vi "Asynchronous Logging Loop.vi"(10 "Input Data":T8 {"File Logging Specs"."File Node Ref" format="%.0x"}) -> ()   [LabVIEW 2027, in "Embedded Data Logger Engine.lvlib"]
uses:
  Embedded Data Logger Engine.lvlib
  File Logging Specification.ctl
  Group Logging Specification.ctl
  Group Buffer Data.ctl
  Property Specification.ctl
  <vilib>/NI VeriStand/Custom Device API/Custom Device Item Ref.ctl
  Shared/Segment Files By.ctl
  Logging State.ctl
  Asynchronous Logging Loop State.ctl
  Add to Flushed Data Size.vi
  Scripting/Embedded Data Logger Scripting.lvlib
  <vilib>/NI VeriStand/Custom Device API/Custom Device API.lvlib
  Shared/Embedded Data Logger Shared.lvlib
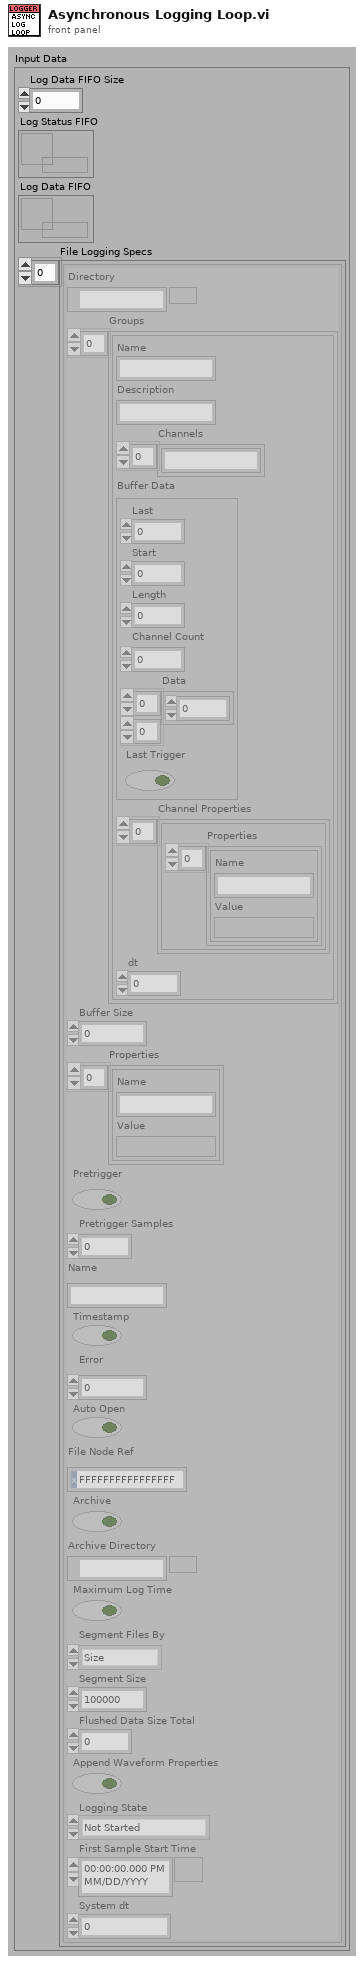
[diagram p1: front panel]
types:
  T1 = typedef "Embedded Data Logger Engine.lvlib/File Logging Specification.ctl" = cluster{"Directory":path, "Groups":T2[], "Buffer Size":i32, "Properties":T4[], "Pretrigger":bool, "Pretrigger Samples":i32, "Name":string, "Timestamp":bool, "Error":i32, "Auto Open":bool, "File Node Ref":T5, "Archive":bool, "Archive Directory":path, "Segment Files":bool, "Segment Files By":T6, "Segment Size":u32, "Flushed Data Size Total":u32, "Append Waveform Properties":bool, "Logging State":T7, "First Sample Start Time":timestamp, "System dt":dbl}
  T2 = typedef "Embedded Data Logger Engine.lvlib/Group Logging Specification.ctl" = cluster{"Name":string, "Description":string, "Channels":string[], "Buffer Data":T3, "Channel Properties":cluster{"Properties":T4[]}[], "dt":dbl}
  T3 = typedef "Embedded Data Logger Engine.lvlib/Group Buffer Data.ctl" = cluster{"Last":i32, "Start":i32, "Length":i32, "Channel Count":i32, "Data":dbl[][], "Last Trigger":bool}
  T4 = typedef "Embedded Data Logger Engine.lvlib/Property Specification.ctl" = cluster{"Name":string, "Value":variant}
  T5 = typedef "Custom Device API.lvlib/Custom Device Item Ref.ctl" = u64
  T6 = typedef "Embedded Data Logger Shared.lvlib/Segment Files By.ctl" = enum16{"Time", "Size"}
  T7 = typedef "Embedded Data Logger Engine.lvlib/Logging State.ctl" = enum16{"Not Started", "Continous Logging", "Paused", "Discontinous Logging"}
  T8 = cluster{"Log Data FIFO Size":i32, "Log Status FIFO":refnum<k33>, "Log Data FIFO":refnum<k33>, "File Logging Specs":T1[]}
  T9 = typedef "Embedded Data Logger Engine.lvlib/Asynchronous Logging Loop State.ctl" = enum16{"Initialize", "Check Cmd", "Log Data", "Open File", "Close File", "Shut Down", "Open File then Log Data"}
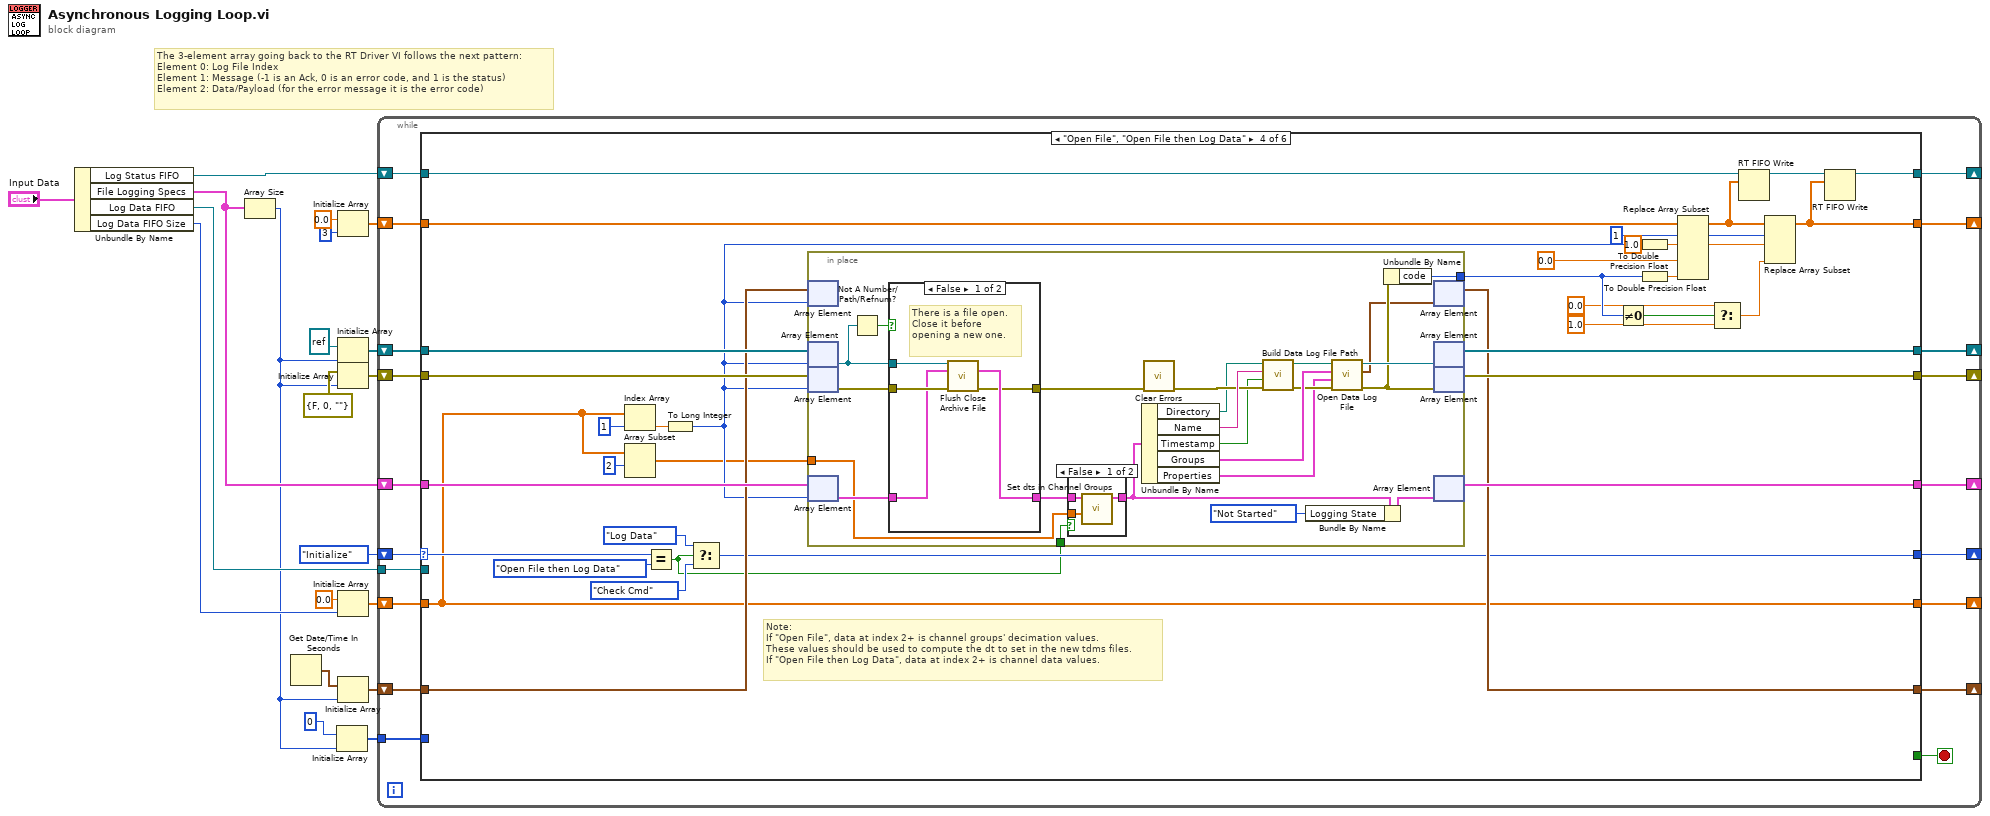
[diagram p0: block diagram]
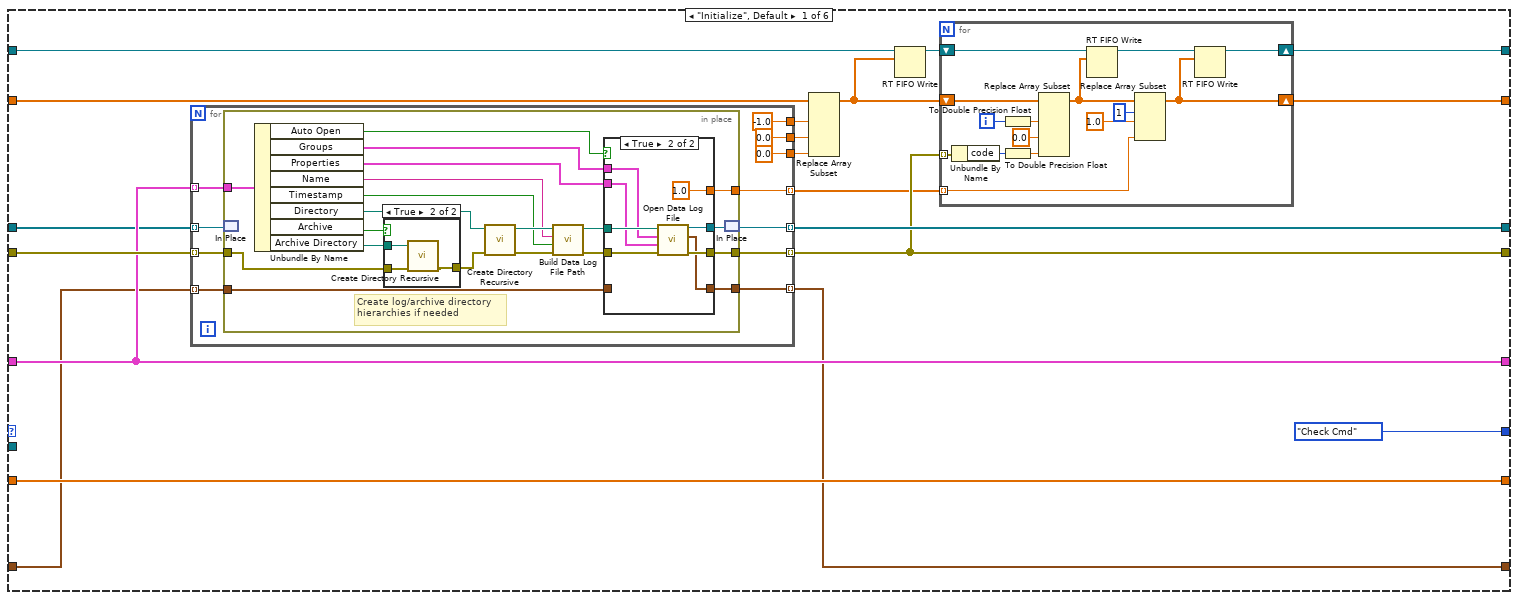
[diagram p2: hidden frame]
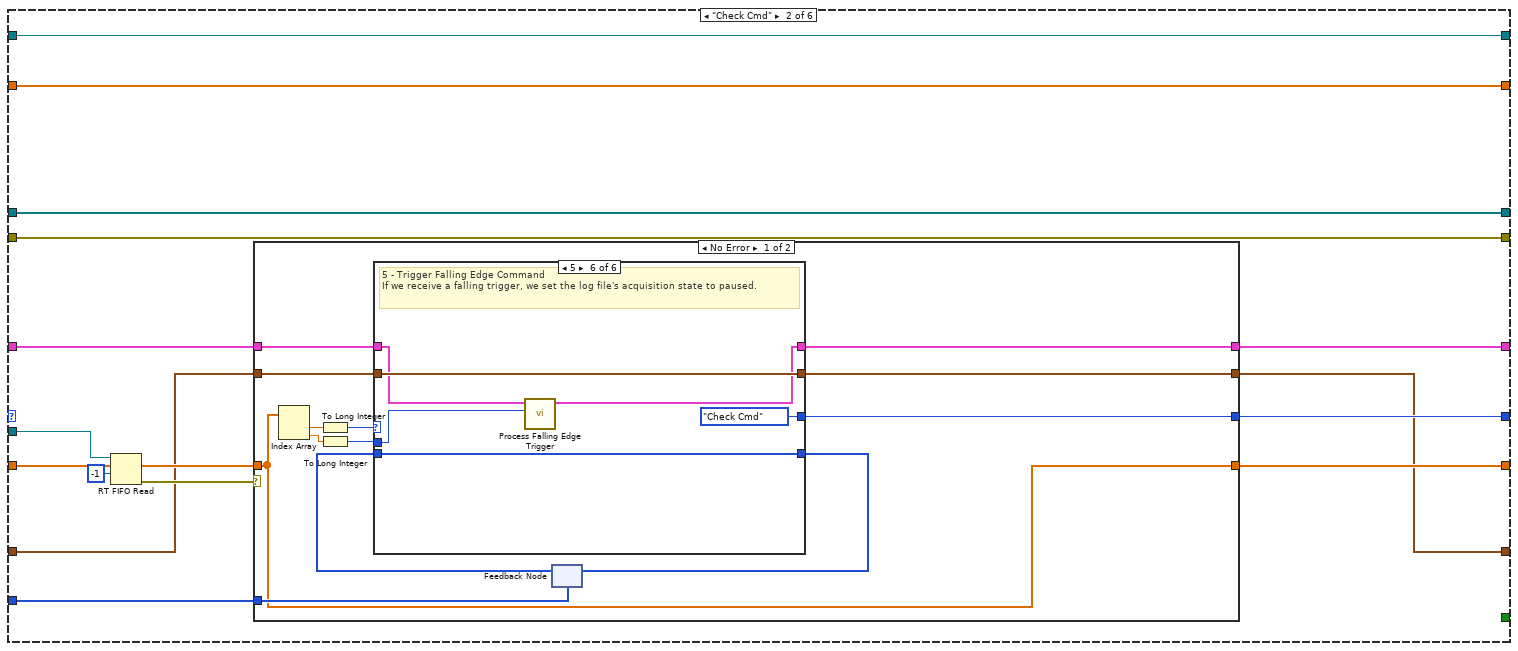
[diagram p5: hidden frame]
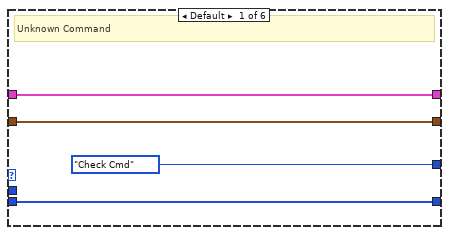
[diagram p6: hidden frame]
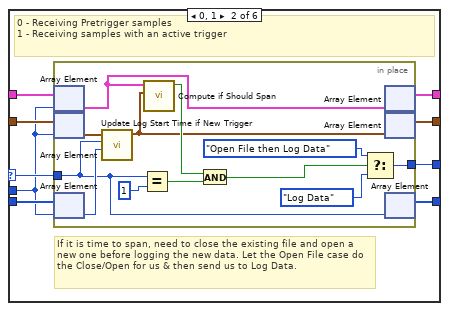
[diagram p7: hidden frame]
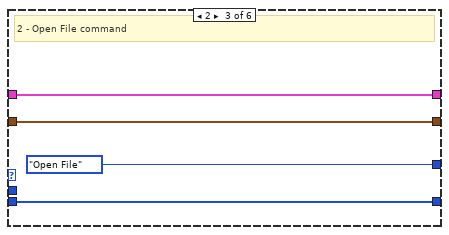
[diagram p8: hidden frame]
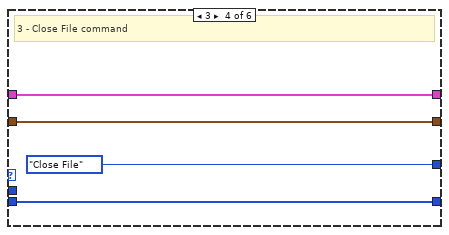
[diagram p9: hidden frame]
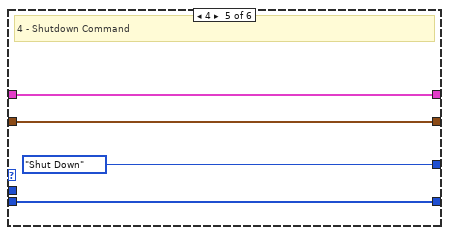
[diagram p10: hidden frame]
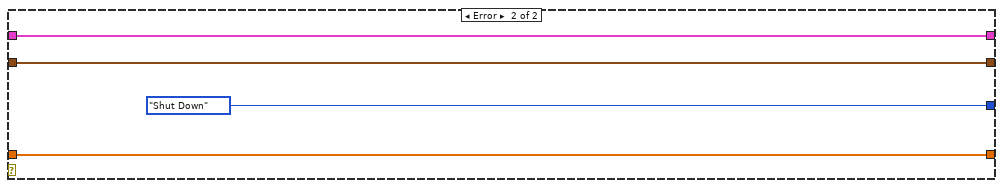
[diagram p11: hidden frame]
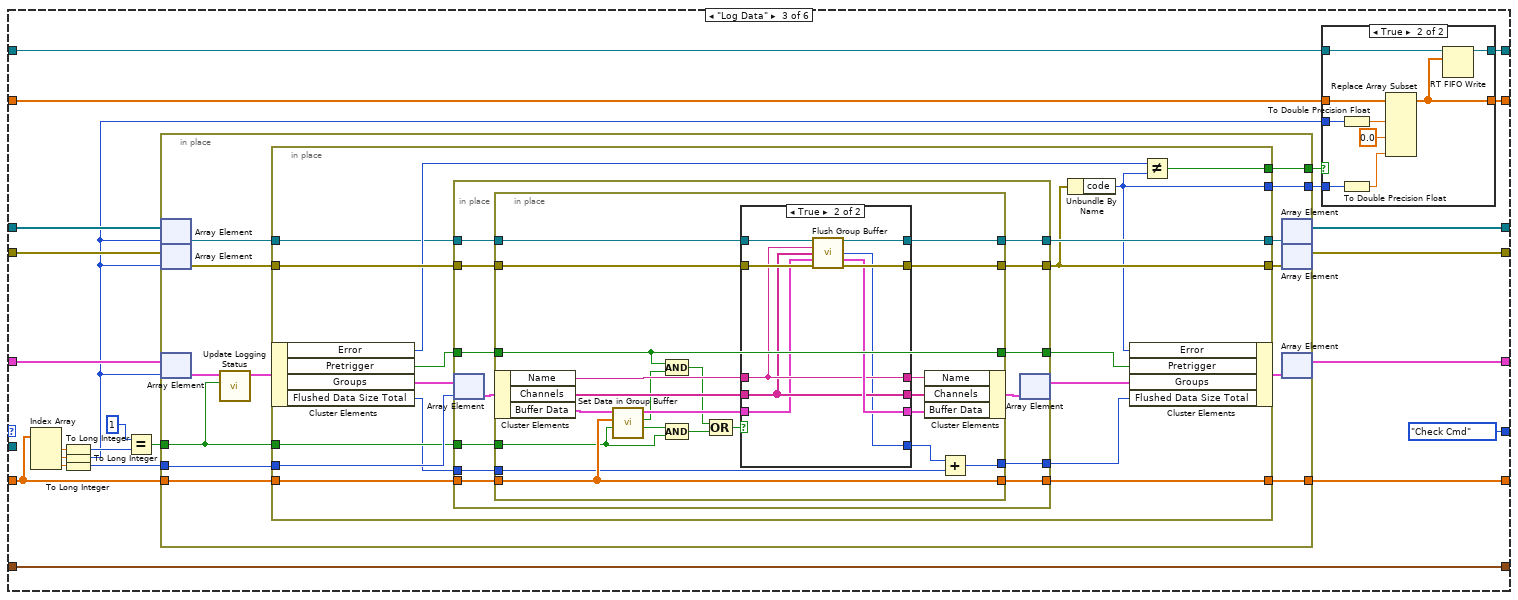
[diagram p12: hidden frame]
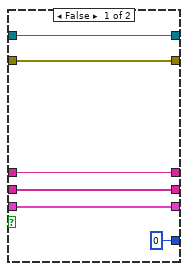
[diagram p13: hidden frame]
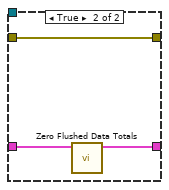
[diagram p16: hidden frame]
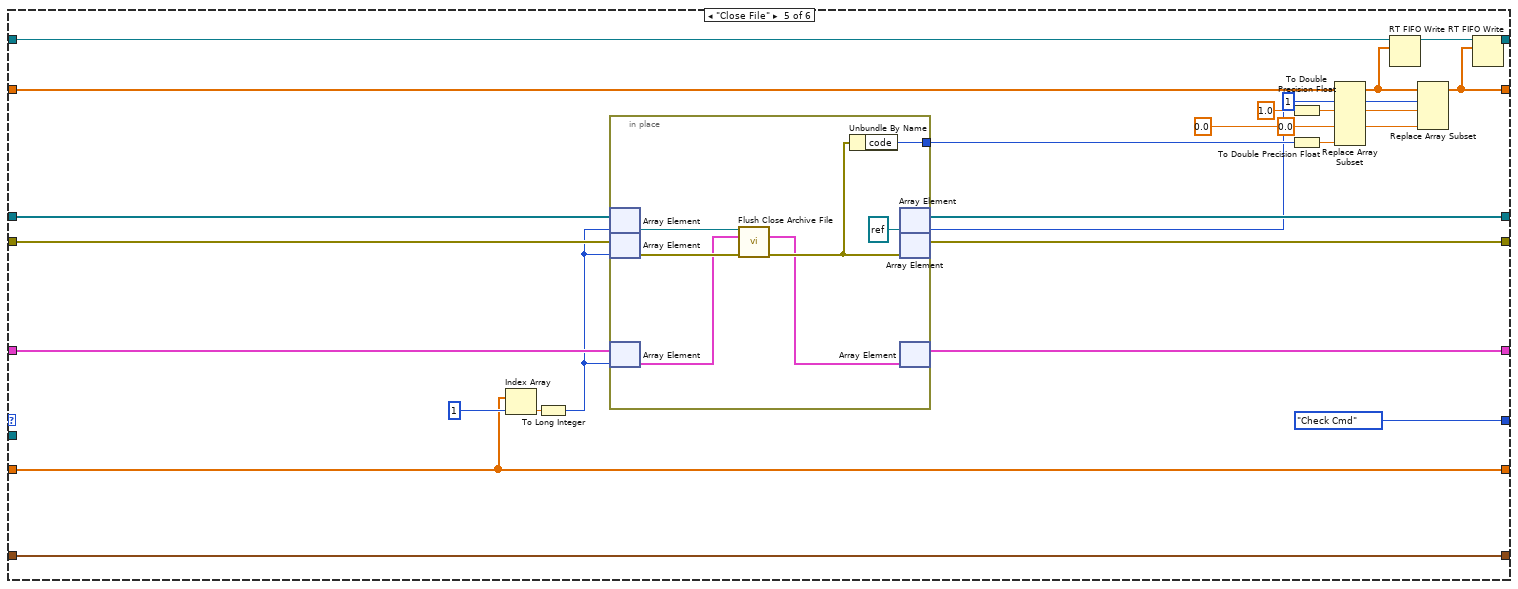
[diagram p17: hidden frame]
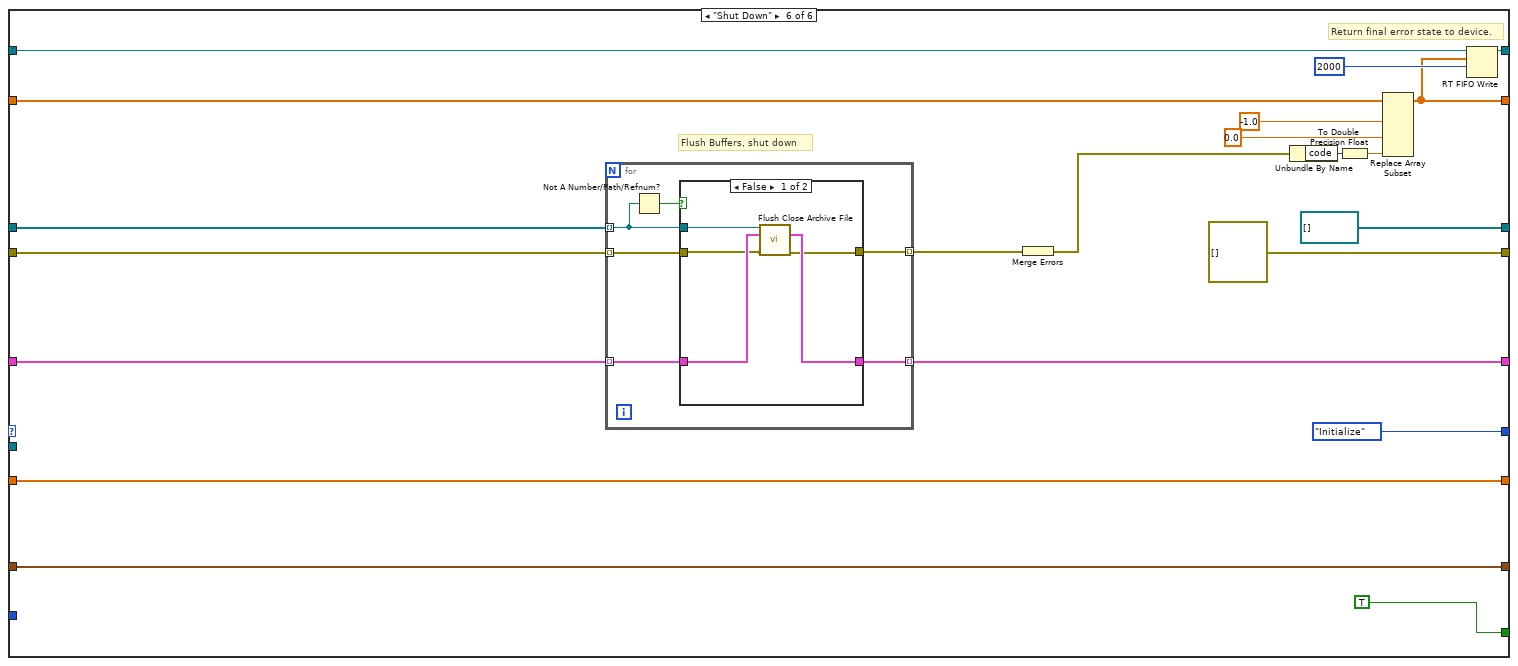
[diagram p18: hidden frame]
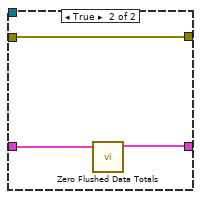
[diagram p19: hidden frame]
diagram:
  # "The 3-element array going back to the RT Driver VI follows the next pattern:\nElement 0: Log File Index\nElement 1: Message (-1 is an Ack, 0 is an error code, and 1 is the status)\nElement 2: Data/Payload (for the error message it is the error code)"
  n1 = Unbundle By Name("Input Data") -> ("Log Status FIFO"=w14:refnum<k33>, "File Logging Specs"=w11:T1[], "Log Data FIFO"=w16:refnum<k33>, "Log Data FIFO Size"=w17:i32)
  n2 = Array Size(array=w11) -> (size(s)=w4:i32)
  n3 = Get Date/Time In Seconds() -> (seconds since 1Jan1904=w1:timestamp)
  n4 = Initialize Array(0 ("y"), w4) -> (w2:i32[])
  n5 = Initialize Array(0.0 ("element"), 3 ("dimension size")) -> (w6:dbl[])
  n6 = Initialize Array(refnum<k34> refnum ("TDMS File Ref out"), w4) -> (w9:refnum<k34>[])
  n7 = Initialize Array(errorcluster {"status"=FALSE, "code"=0, "source"=""} ("error in (no error)"), w4) -> (w12:errorcluster[])
  n8 = Initialize Array(0.0 ("element"), w17) -> (w19:dbl[])
  n9 = Initialize Array(w1, w4) -> (w5:timestamp[])
  n10 = while {
    tunnel: w16 -> [w39]
    shift-right: [w35] -> _
    shift-left: w19 -> [w38]
    shift-right: [w29] -> _
    shift-left: w9 -> [w28]
    shift-right: [w32] -> _
    shift-left: w11 -> [w33]
    shift-right: [w27] -> _
    shift-left: w14 -> [w26]
    shift-right: [w31] -> _
    shift-left: w12 -> [w30]
    shift-right: [w34] -> _
    shift-left: Asynchronous_Logging_Loop_State."Initialize" ("State") -> [w37]
    shift-right: [w24] -> _
    shift-left: w6 -> [w25]
    shift-right: [w22] -> _
    shift-left: w5 -> [w23]
    tunnel: w2 -> [w21]
    stop <- w36 stop-if-true
    n11 = case shown="\"Open File\", \"Open File then Log Data\"" w37 {
      selector: w37 -> [_ _ _ w319 _ _]
      tunnel: w39 -> [_ w134 _ _ _ _]
      tunnel: w38 -> [w57 w120 w213 w312 w399 w431]
      tunnel: [_ _ _ _ _ TRUE] -> w36
      tunnel: [w57 w126 w202 w312 w399 w431] -> w35
      tunnel: [Asynchronous_Logging_Loop_State."Check Cmd" ("State") w125 Asynchronous_Logging_Loop_State."Check Cmd" ("State") w315 Asynchronous_Logging_Loop_State."Check Cmd" ("State") Asynchronous_Logging_Loop_State."Initialize" ("State")] -> w34
      tunnel: w33 -> [w54 w121 w208 w339 w385 w416]
      tunnel: [w54 w122 w203 w338 w382 w415] -> w32
      tunnel: [w51 w130 w204 w340 w401 errorcluster[] []] -> w31
      tunnel: w30 -> [w58 w130 w214 w341 w402 w432]
      tunnel: [w55 w129 w206 w342 w403 refnum<k34>[] []] -> w29
      tunnel: w28 -> [w50 w129 w215 w343 w404 w433]
      tunnel: [w45 w128 w205 w332 w390 w424] -> w27
      tunnel: w26 -> [w53 w128 w218 w334 w397 w417]
      tunnel: w25 -> [w49 w127 w197 w337 w396 w420]
      tunnel: [w44 w127 w198 w330 w386 w421] -> w24
      tunnel: w23 -> [w41 w123 w195 w321 w381 w414]
      tunnel: [w40 w124 w195 w320 w381 w414] -> w22
      tunnel: w21 -> [_ w119 _ _ _ _]
      frame "Initialize", Default {
        n12 = for {
          tunnel: w54 -> [w84] mode=indexing
          tunnel: [w81] -> w55 mode=indexing
          tunnel: [w82] -> w51 mode=indexing
          tunnel: w58 -> [w83] mode=indexing
          tunnel: w50 -> [w80] mode=indexing
          tunnel: [-1.0 ("new element/subarray")] -> w48
          tunnel: [0.0 ("new element/subarray")] -> w47
          tunnel: [w77] -> w43 mode=indexing
          tunnel: [0.0 ("new element/subarray")] -> w42
          tunnel: w41 -> [w74] mode=indexing
          tunnel: [w75] -> w40 mode=indexing
          n13 = in-place {
            in-place-border: w84 -> [w104]
            in-place-border: w83 -> [w90]
            in-place-border: [w96] -> w82
            in-place-border: [w93] -> w77
            in-place-border: [w86] -> w75
            in-place-border: w74 -> [w85]
            # "Create log/archive directory hierarchies if needed"
            n14 = in-place-match #1(w80) -> ()  [unwired: 1 out]
            n15 = Unbundle By Name(w104) -> ("Auto Open"=w94:bool, "Groups"=w97:T2[], "Properties"=w98:T4[], "Name"=w101:string, "Timestamp"=w100:bool, "Directory"=w88:path, "Archive"=w92:bool, "Archive Directory"=w89:path)
            n16 = case shown="True" w92 {
              tunnel: [w105 w108] -> w91
              tunnel: w90 -> [w105 w107]
              tunnel: w89 -> [_ w106]
              frame False {
              }
              frame True {
                n17 = call <vilib>:"Create Directory Recursive.vi"("error in (no error)"=w107, "directory"=w106) -> ("error out"=w108:errorcluster)  [unwired: 1 in, 4 out]
              }
            }
            n18 = call <vilib>:"Create Directory Recursive.vi"("error in (no error)"=w91, "directory"=w88) -> ("error out"=w103:errorcluster, "directory copy"=w102:path)  [unwired: 1 in, 3 out]
            n19 = call "Build Data Log File Path.vi"("error in (no error)"=w103, "Timestamp"=w100, "Name"=w101, "Log File Directory"=w102) -> ("error out"=w99:errorcluster, "appended path"=w87:path)  [unwired: 6 in]
            n20 = case shown="True" w94 {
              tunnel: w99 -> [w110 w118]
              tunnel: w87 -> [_ w117]
              tunnel: w98 -> [_ w116]
              tunnel: w97 -> [_ w115]
              tunnel: [w110 w114] -> w96
              tunnel: [_ w113] -> w95
              tunnel: [_ 1.0 ("new element/subarray")] -> w93
              tunnel: [w109 w111] -> w86
              tunnel: w85 -> [w109 _]
              frame False {
              }
              frame True {
                n21 = call "Open Data Log File.vi"("error in"=w118, "File Properties"=w116, "Channel Groups"=w115, "Data Log File Path"=w117) -> ("error out"=w114:errorcluster, "File Start Time"=w111:timestamp, "tdms file out"=w113:refnum<k34>)  [unwired: 5 in]
              }
            }
            n22 = in-place-match #1(w95) -> (w81:refnum<k34>)
          }
        }
        n23 = Replace Array Subset(array=w49, new element #1=w48, new element #2=w47, new element #3=w42) -> (w46:dbl[])  [unwired: 3 in]
        n24 = RT FIFO Write(0:w53, 1:w46) -> (8:w52:refnum<k33>)  [unwired: 2 in, 4 out]
        n25 = for {
          shift-right: [w63] -> w45
          shift-left: w52 -> [w73]
          tunnel: w51 -> [w71] mode=indexing
          shift-right: [w59] -> w44
          shift-left: w46 -> [w69]
          tunnel: w43 -> [w60] mode=indexing
          i -> [w72]
          n26 = Unbundle By Name(w71) -> ("code"=w70:i32)
          n27 = To Double Precision Float(number=w72) -> (double precision float=w66:dbl)
          n28 = To Double Precision Float(number=w70) -> (double precision float=w68:dbl)
          n29 = Replace Array Subset(array=w69, new element #1=w66, new element #2=0.0 ("new element/subarray"), new element #3=w68) -> (w67:dbl[])  [unwired: 3 in]
          n30 = RT FIFO Write(0:w73, 1:w67) -> (8:w64:refnum<k33>)  [unwired: 2 in, 4 out]
          n31 = Replace Array Subset(array=w67, new element #1=1.0 ("new element/subarray"), index #1=1 ("index"), new element #2=w60) -> (w59:dbl[])  [unwired: 1 in]
          n32 = RT FIFO Write(0:w64, 1:w59) -> (8:w63:refnum<k33>)  [unwired: 2 in, 4 out]
        }
      }
      frame "Check Cmd" {
        n33 = RT FIFO Read(0:w134, 1:w120, 2:-1 ("timeout in ms (0)")) -> (9:w131:dbl[], 11:w132:errorcluster)  [unwired: 1 in, 3 out]
        n34 = case shown="No Error" w132 {
          tunnel: [w135 w193] -> w126
          tunnel: w131 -> [w135 w193]
          tunnel: [w145 Asynchronous_Logging_Loop_State."Shut Down" ("State")] -> w125
          tunnel: w121 -> [w142 w192]
          tunnel: w123 -> [w141 w191]
          tunnel: [w140 w191] -> w124
          tunnel: [w139 w192] -> w122
          tunnel: w119 -> [w138 _]
          frame No Error {
            n35 = Index Array(array=w135) -> (element #1=w147:dbl, element #2=w144:dbl)  [unwired: 2 in]
            n36 = To Long Integer(number=w147) -> (32bit integer=w146:i32)
            n37 = To Long Integer(number=w144) -> (32bit integer=w143:i32)
            n38 = feedback #2(w138) -> (w137:i32[])
            n39 = case shown="5" w146 {
              selector: w146 -> [_ w155 _ _ _ _]
              tunnel: [Asynchronous_Logging_Loop_State."Check Cmd" ("State") w158 Asynchronous_Logging_Loop_State."Open File" ("State") Asynchronous_Logging_Loop_State."Close File" ("State") Asynchronous_Logging_Loop_State."Shut Down" ("State") Asynchronous_Logging_Loop_State."Check Cmd" ("State")] -> w145
              tunnel: w143 -> [_ w153 _ _ _ w186]
              tunnel: w142 -> [w149 w160 w174 w178 w182 w188]
              tunnel: w141 -> [w150 w159 w176 w179 w183 w190]
              tunnel: [w150 w157 w176 w179 w183 w190] -> w140
              tunnel: [w149 w156 w174 w178 w182 w187] -> w139
              tunnel: w137 -> [w148 w154 w175 w177 w181 w189]
              tunnel: [w148 w152 w175 w177 w181 w189] -> w136
              frame Default {
                # "Unknown Command"
              }
              frame 0, 1 {
                # "If it is time to span, need to close the existing file and open a new one before logging the new data. Let the Open File case do the Close/Open for us & then send us to Log Data."
                # "0 - Receiving Pretrigger samples\n1 - Receiving samples with an active trigger"
                n40 = in-place {
                  in-place-border: [w170] -> w158
                  in-place-border: w155 -> [w161]
                  n41 = in-place-array #3(w160, w153) -> (w169:T1)
                  n42 = in-place-array #4(w159, w153) -> (w166:timestamp)
                  n43 = in-place-array #5(w154, w153) -> (w162:i32)
                  n44 = call "Update Log Start Time if New Trigger.vi"("Previous Trigger Value"=w162, "Current Trigger Value"=w161, "Previous Log Trigger Time"=w166) -> ("Current Log Trigger Time"=w165:timestamp)  [unwired: 8 in]
                  n45 = Equal?(x=w161, y=1) -> (x = y?=w163:bool)
                  n46 = call "Compute if Should Span.vi"("Log Start Time"=w165, "File Log Specification"=w169) -> ("Span File"=w168:bool)  [unwired: 9 in]
                  n47 = And(x=w168, y=w163) -> (x .and. y?=w167:bool)
                  n48 = Select(t=Asynchronous_Logging_Loop_State."Open File then Log Data" ("State"), s=w167, f=Asynchronous_Logging_Loop_State."Log Data" ("State")) -> (s? t:f=w170:T9)
                  n49 = in-place-array #3(w169) -> (w156:T1[])  [unwired: 1 out]
                  n50 = in-place-array #4(w165) -> (w157:timestamp[])  [unwired: 1 out]
                  n51 = in-place-array #5(w161) -> (w152:i32[])  [unwired: 1 out]
                }
              }
              frame 2 {
                # "2 - Open File command"
              }
              frame 3 {
                # "3 - Close File command"
              }
              frame 4 {
                # "4 - Shutdown Command"
              }
              frame 5 {
                # "5 - Trigger Falling Edge Command\nIf we receive a falling trigger, we set the log file's acquisition state to paused."
                n52 = call "Process Falling Edge Trigger.vi"("Log File Index"=w186, "File Logging Specs in"=w188) -> ("File Logging Specs out"=w187:T1[])  [unwired: 9 in]
              }
            }
            n53 = feedback-in #2(w136) -> ()
          }
          frame Error {
          }
        }
      }
      frame "Log Data" {
        n54 = Index Array(array=w213) -> (element #1=w212:dbl, element #2=w211:dbl, element #3=w210:dbl)  [unwired: 3 in]
        n55 = To Long Integer(number=w212) -> (32bit integer=w209:i32)
        n56 = To Long Integer(number=w211) -> (32bit integer=w196:i32)
        n57 = To Long Integer(number=w210) -> (32bit integer=w207:i32)
        n58 = Equal?(x=1, y=w209) -> (x = y?=w216:bool)
        n59 = in-place {
          in-place-border: w213 -> [w231]
          in-place-border: w207 -> [w230]
          in-place-border: w216 -> [w219]
          in-place-border: [w226] -> w202
          in-place-border: [w223] -> w200
          in-place-border: [w222] -> w199
          n60 = in-place-array #6(w215, w196) -> (w228:refnum<k34>)
          n61 = in-place-array #7(w214, w196) -> (w225:errorcluster)
          n62 = in-place-array #8(w208, w196) -> (w229:T1)
          n63 = call "Update Logging Status.vi"("Log File Trigger"=w219, "File Log Spec in"=w229) -> ("File Log Spec out"=w220:T1)  [unwired: 9 in]
          n64 = in-place {
            in-place-border: w231 -> [w246]
            in-place-border: w230 -> [w245]
            in-place-border: w219 -> [w242]
            in-place-border: w225 -> [w248]
            in-place-border: [w236] -> w224
            in-place-border: w228 -> [w241]
            in-place-border: [w240] -> w227
            in-place-border: [w239] -> w226
            in-place-border: [w235] -> w223
            in-place-border: [w234] -> w222
            n65 = in-place-cluster #9(w220) -> ("Error"=w247:i32, "Pretrigger"=w238:bool, "Groups"=w244:T2[], "Flushed Data Size Total"=w233:u32)
            n66 = in-place {
              in-place-border: w246 -> [w261]
              in-place-border: w242 -> [w249]
              in-place-border: w248 -> [w258]
              in-place-border: [w257] -> w236
              in-place-border: w241 -> [w256]
              in-place-border: [w255] -> w240
              in-place-border: [w254] -> w239
              in-place-border: w238 -> [w253]
              in-place-border: [w252] -> w237
              in-place-border: w233 -> [w251]
              in-place-border: [w250] -> w232
              n67 = in-place-array #10(w244, w245) -> (w260:T2)
              n68 = in-place {
                in-place-border: w261 -> [w271]
                in-place-border: w249 -> [w270]
                in-place-border: w258 -> [w283]
                in-place-border: [w277] -> w257
                in-place-border: w256 -> [w272]
                in-place-border: [w273] -> w255
                in-place-border: [w271] -> w254
                in-place-border: w253 -> [w266]
                in-place-border: [w266] -> w252
                in-place-border: w251 -> [w264]
                in-place-border: [w263] -> w250
                n69 = in-place-cluster #11(w260) -> ("Name"=w278:string, "Channels"=w276:string[], "Buffer Data"=w282:T3)
                n70 = call "Set Data in Group Buffer.vi"("New Trigger"=w270, "Data in"=w271, "Group Buffer Data in"=w282) -> ("Buffer Full"=w281:bool, "Flush Pretrigger Data"=w269:bool, "Group Buffer Data out"=w279:T3)  [unwired: 6 out]
                n71 = Compound Arithmetic op=AND(w266, w269) -> (w267:bool)
                n72 = Compound Arithmetic op=AND(w281, w270) -> (w280:bool)
                n73 = Compound Arithmetic op=OR(w267, w280) -> (w268:bool)
                n74 = case shown="True" w268 {
                  tunnel: w279 -> [w289 w291]
                  tunnel: w278 -> [w287 w293]
                  tunnel: [w289 w296] -> w265
                  tunnel: w283 -> [w288 w298]
                  tunnel: [w288 w297] -> w277
                  tunnel: w276 -> [w286 w292]
                  tunnel: [w287 w293] -> w275
                  tunnel: [w286 w292] -> w274
                  tunnel: [w285 w294] -> w273
                  tunnel: w272 -> [w285 w295]
                  tunnel: [u32 0 ("Flushed Data Size") w290] -> w262
                  frame False {
                  }
                  frame True {
                    n75 = call "Flush Group Buffer.vi"("TDMS File Ref in"=w295, "Group Name"=w293, "Channels"=w292, "Group Buffer Data in"=w291, "error in (no error)"=w298) -> ("TDMS File Ref out"=w294:refnum<k34>, "Flushed Data Size"=w290:u32, "Group Buffer Data out"=w296:T3, "error out"=w297:errorcluster)  [unwired: 1 in, 6 out]
                  }
                }
                n76 = in-place-cluster #11("Name"=w275, "Channels"=w274, "Buffer Data"=w265) -> (w259:T2)
                n77 = Add(x=w262, y=w264) -> (x+y=w263:u32)
              }
              n78 = in-place-array #10(w259) -> (w243:T2[])  [unwired: 1 out]
            }
            n79 = Unbundle By Name(w236) -> ("code"=w235:i32)
            n80 = in-place-cluster #9("Error"=w235, "Pretrigger"=w237, "Groups"=w243, "Flushed Data Size Total"=w232) -> (w221:T1)
            n81 = Not Equal?(x=w247, y=w235) -> (x != y?=w234:bool)
          }
          n82 = in-place-array #6(w227) -> (w206:refnum<k34>[])  [unwired: 1 out]
          n83 = in-place-array #7(w224) -> (w204:errorcluster[])  [unwired: 1 out]
          n84 = in-place-array #8(w221) -> (w203:T1[])  [unwired: 1 out]
        }
        n85 = case shown="True" w199 {
          tunnel: w218 -> [w300 w309]
          tunnel: w196 -> [_ w308]
          tunnel: [w300 w307] -> w205
          tunnel: w200 -> [_ w306]
          tunnel: [w299 w304] -> w198
          tunnel: w197 -> [w299 w305]
          frame False {
          }
          frame True {
            n86 = To Double Precision Float(number=w308) -> (double precision float=w302:dbl)
            n87 = To Double Precision Float(number=w306) -> (double precision float=w303:dbl)
            n88 = Replace Array Subset(array=w305, new element #1=w302, new element #2=0.0 ("new element/subarray"), new element #3=w303) -> (w304:dbl[])  [unwired: 3 in]
            n89 = RT FIFO Write(0:w309, 1:w304) -> (8:w307:refnum<k33>)  [unwired: 2 in, 4 out]
          }
        }
      }
      frame "Open File", "Open File then Log Data" {
        # "Note:\nIf \"Open File\", data at index 2+ is channel groups' decimation values.\nThese values should be used to compute the dt to set in the new tdms files.\nIf \"Open File then Log Data\", data at index 2+ is channel data values."
        n90 = Index Array(array=w312, index=1) -> (element=w345:dbl)
        n91 = Array Subset(array=w312, index=2) -> (w311:dbl[])  [unwired: 1 in]
        n92 = Equal?(x=w319, y=Asynchronous_Logging_Loop_State."Open File then Log Data" ("State")) -> (x = y?=w310:bool)
        n93 = To Long Integer(number=w345) -> (32bit integer=w314:i32)
        n94 = Select(t=Asynchronous_Logging_Loop_State."Log Data" ("State"), s=w310, f=Asynchronous_Logging_Loop_State."Check Cmd" ("State")) -> (s? t:f=w315:T9)
        n95 = in-place {
          in-place-border: [w362] -> w326
          in-place-border: w311 -> [w349]
          in-place-border: w310 -> [w346]
          n96 = in-place-array #12(w321, w314) -> ()  [unwired: 1 out]
          n97 = in-place-array #13(w343, w314) -> (w357:refnum<k34>)
          n98 = in-place-array #14(w341, w314) -> (w364:errorcluster)
          n99 = in-place-array #15(w339, w314) -> (w355:T1)
          n100 = Not A Number/Path/Refnum?(number/path/refnum=w357) -> (NaN/Path/Refnum?=w356:bool)
          n101 = case shown="False" w356 {
            tunnel: w364 -> [w376 w380]
            tunnel: [w373 w380] -> w363
            tunnel: w357 -> [w377 _]
            tunnel: [w374 w378] -> w348
            tunnel: w355 -> [w375 w379]
            frame False {
              # "There is a file open. Close it before opening a new one."
              n102 = call "Flush Close Archive File.vi"("TDMS File Refnum In"=w377, "File Log Spec In"=w375, "error in"=w376) -> ("File Log Spec Out"=w374:T1, "error out"=w373:errorcluster)  [unwired: 11 in]
            }
            frame True {
              n103 = call "Zero Flushed Data Totals.vi"("File Log Spec in"=w379) -> ("File Log Spec out"=w378:T1)  [unwired: 10 in]
            }
          }
          n104 = case shown="False" w346 {
            tunnel: w349 -> [w371 _]
            tunnel: w348 -> [w370 w372]
            tunnel: [w369 w372] -> w347
            frame False {
              n105 = call "Set dts in Channel Groups.vi"("channel groups decimations"=w371, "File Log Spec in"=w370) -> ("File Log Spec out"=w369:T1)  [unwired: 8 in, 1 out]
            }
            frame True {
            }
          }
          n106 = Unbundle By Name(w347) -> ("Directory"=w360:path, "Name"=w368:string, "Timestamp"=w359:bool, "Groups"=w367:T2[], "Properties"=w358:T4[])
          n107 = call <vilib>:"Clear Errors.vi"("error in (no error)"=w363) -> ("error out"=w361:errorcluster)  [unwired: 5 in, 1 out]
          n108 = call "Build Data Log File Path.vi"("error in (no error)"=w361, "Timestamp"=w359, "Name"=w368, "Log File Directory"=w360) -> ("error out"=w366:errorcluster, "appended path"=w354:path)  [unwired: 6 in]
          n109 = Bundle By Name(cluster=w347, "Logging State"=Logging_State."Not Started") -> (w351:T1)
          n110 = call "Open Data Log File.vi"("error in"=w366, "File Properties"=w358, "Channel Groups"=w367, "Data Log File Path"=w354) -> ("error out"=w353:errorcluster, "File Start Time"=w352:timestamp, "tdms file out"=w365:refnum<k34>)  [unwired: 5 in]
          n111 = Unbundle By Name(w353) -> ("code"=w362:i32)
          n112 = in-place-array #12(w352) -> (w320:timestamp[])  [unwired: 1 out]
          n113 = in-place-array #13(w365) -> (w342:refnum<k34>[])  [unwired: 1 out]
          n114 = in-place-array #14(w353) -> (w340:errorcluster[])  [unwired: 1 out]
          n115 = in-place-array #15(w351) -> (w338:T1[])  [unwired: 1 out]
        }
        n116 = Not Equal To 0?(x=w326) -> (x != 0?=w325:bool)
        n117 = To Double Precision Float(number=w314) -> (double precision float=w329:dbl)
        n118 = To Double Precision Float(number=w326) -> (double precision float=w336:dbl)
        n119 = Replace Array Subset(array=w337, new element #1=w329, new element #2=0.0 ("new element/subarray"), new element #3=w336) -> (w331:dbl[])  [unwired: 3 in]
        n120 = Select(t=0.0, s=w325, f=1.0 ("new element/subarray")) -> (s? t:f=w322:dbl)
        n121 = RT FIFO Write(0:w334, 1:w331) -> (8:w333:refnum<k33>)  [unwired: 2 in, 4 out]
        n122 = Replace Array Subset(array=w331, new element #1=1.0 ("new element/subarray"), index #1=1 ("index"), new element #2=w322) -> (w330:dbl[])  [unwired: 1 in]
        n123 = RT FIFO Write(0:w333, 1:w330) -> (8:w332:refnum<k33>)  [unwired: 2 in, 4 out]
      }
      frame "Close File" {
        n124 = Index Array(array=w399, index=1) -> (element=w406:dbl)
        n125 = To Long Integer(number=w406) -> (32bit integer=w384:i32)
        n126 = in-place {
          in-place-border: [w413] -> w398
          n127 = in-place-array #16(w404, w384) -> (w410:refnum<k34>)
          n128 = in-place-array #17(w402, w384) -> (w411:errorcluster)
          n129 = in-place-array #18(w385, w384) -> (w409:T1)
          n130 = call "Flush Close Archive File.vi"("TDMS File Refnum In"=w410, "File Log Spec In"=w409, "error in"=w411) -> ("File Log Spec Out"=w407:T1, "error out"=w408:errorcluster)  [unwired: 11 in]
          n131 = Unbundle By Name(w408) -> ("code"=w413:i32)
          n132 = in-place-array #16(refnum<k34> refnum ("element")) -> (w403:refnum<k34>[], w383:i32)
          n133 = in-place-array #17(w408) -> (w401:errorcluster[])  [unwired: 1 out]
          n134 = in-place-array #18(w407) -> (w382:T1[])  [unwired: 1 out]
        }
        n135 = To Double Precision Float(number=w383) -> (double precision float=w393:dbl)
        n136 = To Double Precision Float(number=w398) -> (double precision float=w394:dbl)
        n137 = Replace Array Subset(array=w396, new element #1=w393, new element #2=0.0 ("new element/subarray"), new element #3=w394) -> (w395:dbl[])  [unwired: 3 in]
        n138 = RT FIFO Write(0:w397, 1:w395) -> (8:w391:refnum<k33>)  [unwired: 2 in, 4 out]
        n139 = Replace Array Subset(array=w395, new element #1=1.0 ("new element/subarray"), index #1=1 ("index"), new element #2=0.0 ("new element/subarray")) -> (w386:dbl[])  [unwired: 1 in]
        n140 = RT FIFO Write(0:w391, 1:w386) -> (8:w390:refnum<k33>)  [unwired: 2 in, 4 out]
      }
      frame "Shut Down" {
        # "Return final error state to device."
        # "Flush Buffers, shut down"
        n141 = for {
          tunnel: w416 -> [w439] mode=indexing
          tunnel: w433 -> [w437] mode=indexing
          tunnel: w432 -> [w440] mode=indexing
          tunnel: [w438] -> w423 mode=indexing
          tunnel: [w435] -> w415 mode=indexing
          n142 = Not A Number/Path/Refnum?(number/path/refnum=w437) -> (NaN/Path/Refnum?=w436:bool)
          n143 = case shown="False" w436 {
            tunnel: w440 -> [w443 w448]
            tunnel: w439 -> [w444 w447]
            tunnel: [w441 w448] -> w438
            tunnel: w437 -> [w445 _]
            tunnel: [w442 w446] -> w435
            frame False {
              n144 = call "Flush Close Archive File.vi"("TDMS File Refnum In"=w445, "File Log Spec In"=w444, "error in"=w443) -> ("File Log Spec Out"=w442:T1, "error out"=w441:errorcluster)  [unwired: 11 in]
            }
            frame True {
              n145 = call "Zero Flushed Data Totals.vi"("File Log Spec in"=w447) -> ("File Log Spec out"=w446:T1)  [unwired: 10 in]
            }
          }
        }
        n146 = Merge Errors(w423) -> (w422:errorcluster)
        n147 = Unbundle By Name(w422) -> ("code"=w425:i32)
        n148 = To Double Precision Float(number=w425) -> (double precision float=w428:dbl)
        n149 = Replace Array Subset(array=w420, new element #1=-1.0 ("new element/subarray"), new element #2=0.0 ("new element/subarray"), new element #3=w428) -> (w421:dbl[])  [unwired: 3 in]
        n150 = RT FIFO Write(0:w417, 1:w421, 2:2000 ("timeout in ms (0)")) -> (8:w424:refnum<k33>)  [unwired: 2 in, 3 out]
      }
    }
  }
